vi "rszvl Query OPC.vi"(8 "error in (no error)":errorcluster, 11 "VISA resource name":refnum<visa-resource-name>) -> (0 "error out":errorcluster, 2 "OPC":i32, 3 "VISA resource name out":refnum<visa-resource-name>)   [LabVIEW 2014]
doc: "This VI sends OPC query to the instrument. This effectively causes your program to wait in this VI until the instrument has processed all the commands you have sent to it until this point. Use the VI to force the synchronization of the instrument with you program.\n\nAttribute(s):\n-\n\nRemote-control command(s):\n*OPC?"
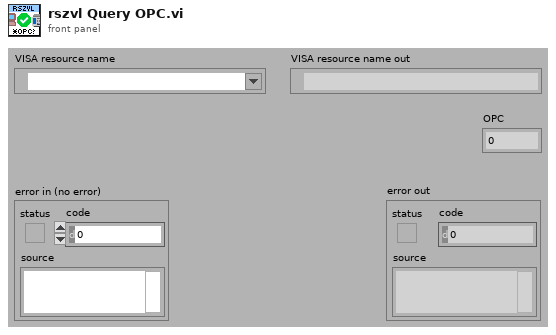
[diagram p1: front panel]
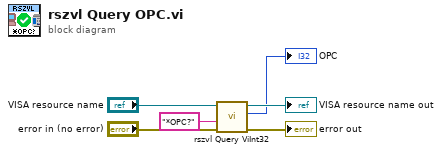
[diagram p0: block diagram]
diagram:
  n1 = call "rszvl Query ViInt32.vi"("error in (no error)"="error in (no error)", "Command"="*OPC?" ("Revision Query Command"), "VISA resource name"="VISA resource name") -> ("error out"=→"error out":errorcluster, "Value"=→"OPC":i32, "VISA resource name out"=→"VISA resource name out":refnum<visa-resource-name>)  [unwired: 6 in]
